vi "Servo_serial_mac_readwrite.vi"() -> ()   [LabVIEW 2017]
uses:
  <vilib>/Instr/_visa.llb/VISA Configure Serial Port (Instr).vi
panel:
  out "Servo 5 Position":cluster{i32, dbl, dbl[][]}(graph)
  out "Servo 4 Position":cluster{i32, dbl, dbl[][]}(graph)
  out "Servo 3 Position":cluster{i32, dbl, dbl[][]}(graph)
  out "Servo 2 Position":cluster{i32, dbl, dbl[][]}(graph)
  out "Servo 1 Position":cluster{i32, dbl, dbl[][]}(graph)
  out "Pos1 number":dbl
  out "Pos2 number":dbl
  out "Pos3 number":dbl
  out "Pos4 number":dbl
  out "Pos5 number":dbl
  in  "Delay":dbl
  in  "Buad Rate":i32(ring) items=["2400"=2400, "4800"=4800, "9600"=9600, "14400"=14400, "19200"=19200, "28800"=28800, "38400"=38400, "57600"=57600, "115200"=115200]
  out "Bytes at port":cluster{i32, dbl, dbl[]}(graph)
  out "Read from Arduino":string
  in  "Servo 5":dbl(knob) scale=0.0..180.0
  in  "Servo 4":dbl(knob) scale=0.0..180.0
  in  "Servo 3":dbl(knob) scale=0.0..180.0
  in  "Servo 2":dbl(knob) scale=0.0..180.0
  in  "Servo 1":dbl(knob) scale=0.0..180.0
  in  "stop":bool
  out "Sent to Arduino":string
  in  "COM Port":refnum<visa-resource-name>
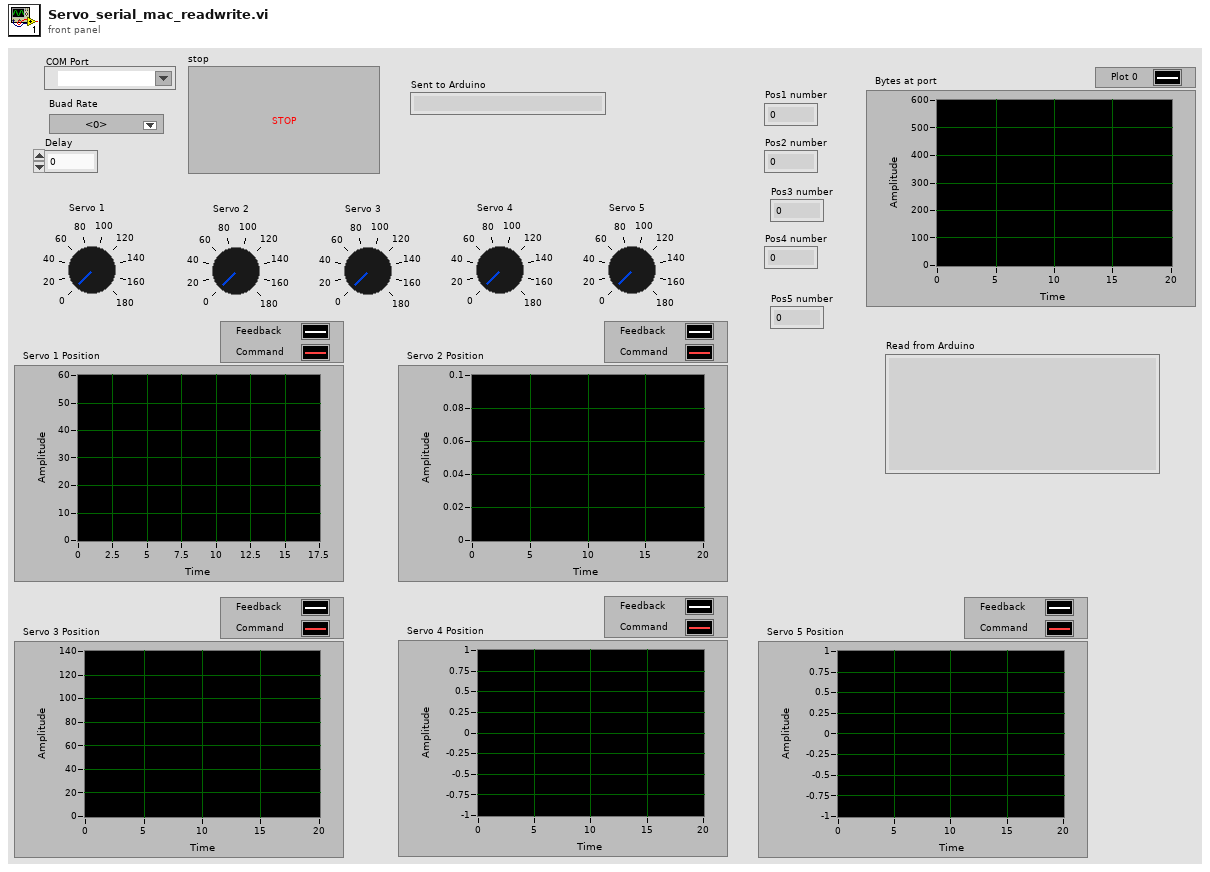
[diagram p1: front panel]
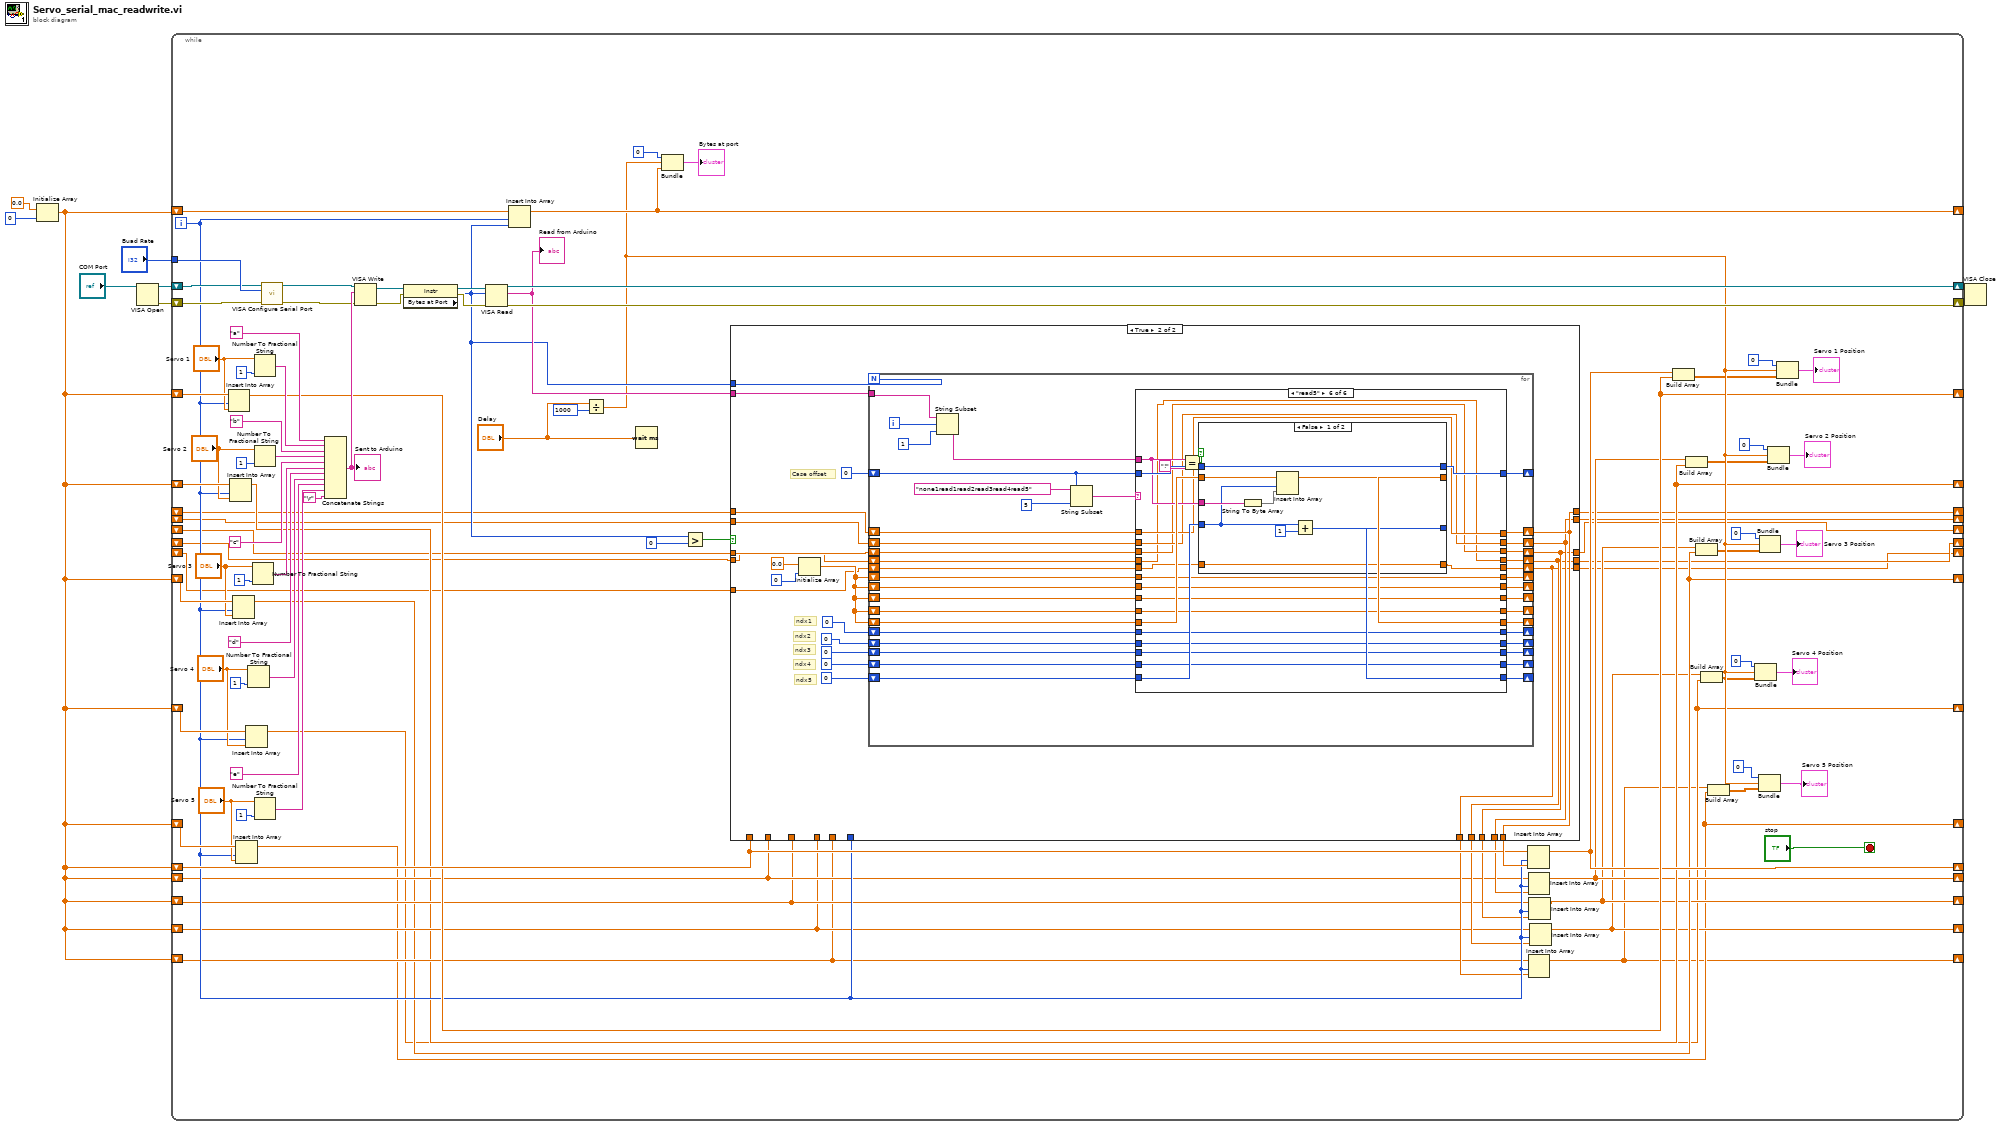
[diagram p0: block diagram]
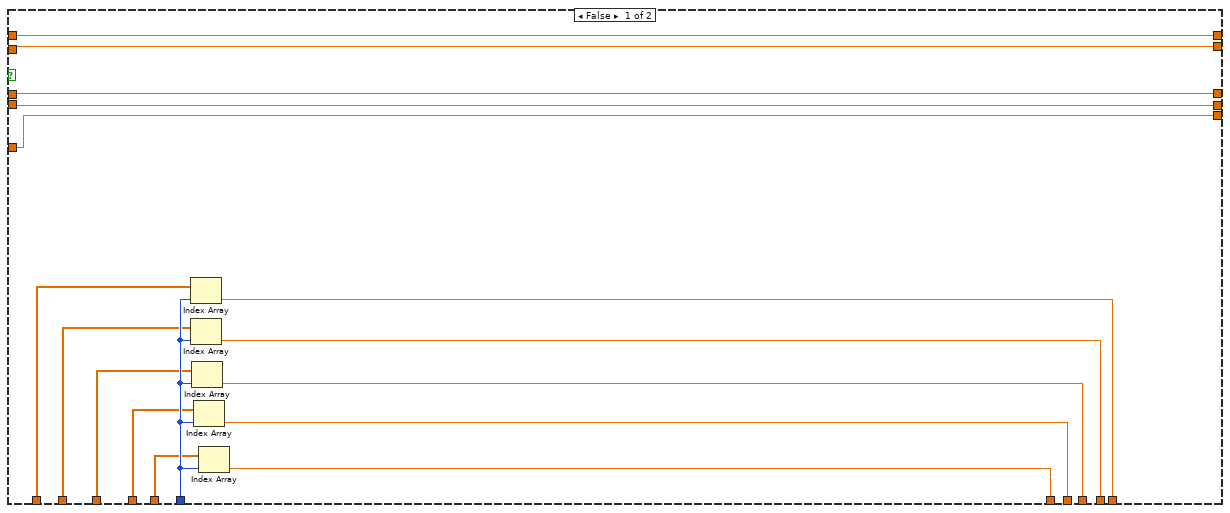
[diagram p2: hidden frame]
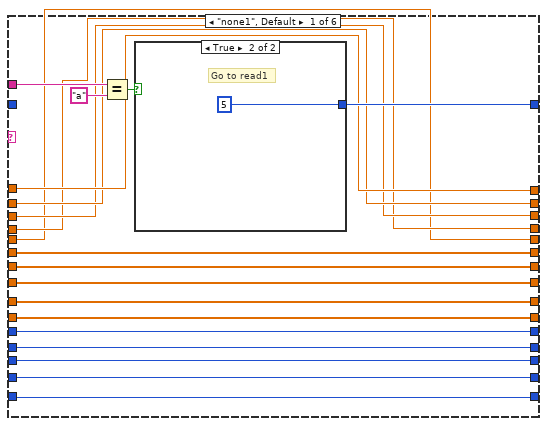
[diagram p3: hidden frame]
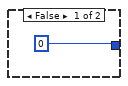
[diagram p4: hidden frame]
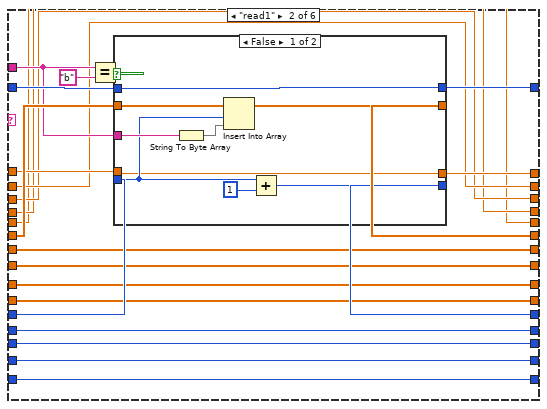
[diagram p5: hidden frame]
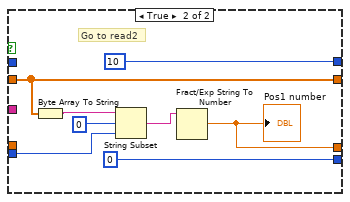
[diagram p6: hidden frame]
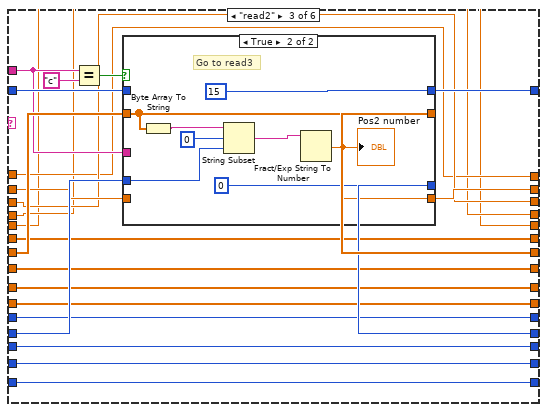
[diagram p7: hidden frame]
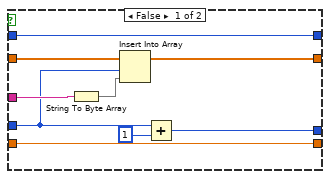
[diagram p8: hidden frame]
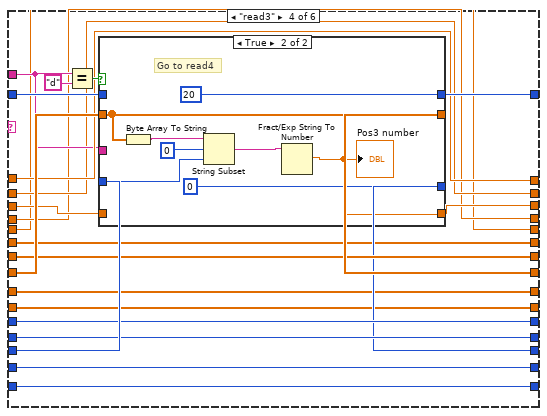
[diagram p9: hidden frame]
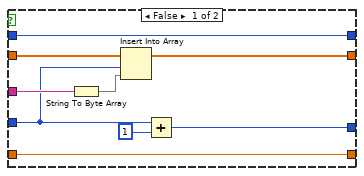
[diagram p10: hidden frame]
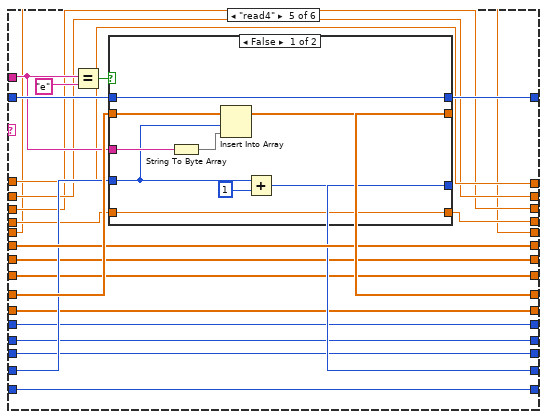
[diagram p11: hidden frame]
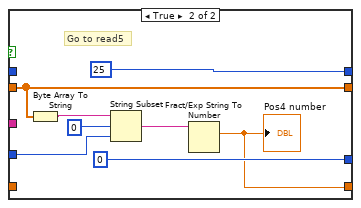
[diagram p12: hidden frame]
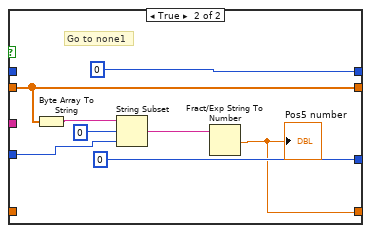
[diagram p13: hidden frame]
diagram:
  n1 = Initialize Array(0.0 ("element"), 0 ("dimension size")) -> (w1:dbl[])
  n2 = VISA Open(VISA resource name="COM Port") -> (VISA resource name=w8:refnum<visa-resource-name>, error out=w7:errorcluster)  [unwired: 4 in]
  n3 = while {
    tunnel: "Buad Rate" -> [w105]
    shift-right: [w101] -> w6
    shift-left: w8 -> [w104]
    shift-right: [w102] -> w5
    shift-left: w7 -> [w103]
    shift-right: [w99] -> _
    shift-left: w1 -> [w100]
    shift-right: [w43] -> _
    shift-left: w1 -> [w66]
    shift-right: [w30] -> _
    shift-left: w1 -> [w65]
    shift-right: [w27] -> _
    shift-left: w1 -> [w64]
    shift-right: [w24] -> _
    shift-left: w1 -> [w63]
    shift-right: [w21] -> _
    shift-left: w1 -> [w62]
    shift-right: [w41] -> _
    shift-left: w1 -> [w45]
    shift-right: [w29] -> _
    shift-left: w1 -> [w35]
    shift-right: [w26] -> _
    shift-left: w1 -> [w34]
    shift-right: [w23] -> _
    shift-left: w1 -> [w33]
    shift-right: [w20] -> _
    shift-left: w1 -> [w32]
    shift-right: [w18] -> _
    shift-left: _ -> [w19]
    shift-right: [w13] -> _
    shift-left: _ -> [w17]
    shift-right: [w12] -> _
    shift-left: _ -> [w16]
    shift-right: [w11] -> _
    shift-left: _ -> [w15]
    shift-right: [w10] -> _
    shift-left: _ -> [w14]
    i -> [w40]
    stop <- "stop" stop-if-true
    n4 = Insert Into Array(array=w66, index=w40, new element="Servo 1") -> (w43:dbl[])
    n5 = Insert Into Array(array=w65, index=w40, new element="Servo 2") -> (w30:dbl[])
    n6 = Insert Into Array(array=w64, index=w40, new element="Servo 3") -> (w27:dbl[])
    n7 = Insert Into Array(array=w62, index=w40, new element="Servo 5") -> (w21:dbl[])
    n8 = Insert Into Array(array=w63, index=w40, new element="Servo 4") -> (w24:dbl[])
    n9 = Number To Fractional String(number="Servo 4", precision (6)=1) -> (F-format string=w86:string)  [unwired: 2 in]
    n10 = Number To Fractional String(number="Servo 3", precision (6)=1) -> (F-format string=w93:string)  [unwired: 2 in]
    n11 = Number To Fractional String(number="Servo 1", precision (6)=1) -> (F-format string=w95:string)  [unwired: 2 in]
    n12 = Number To Fractional String(number="Servo 2", precision (6)=1) -> (F-format string=w94:string)  [unwired: 2 in]
    n13 = Number To Fractional String(number="Servo 5", precision (6)=1) -> (F-format string=w85:string)  [unwired: 2 in]
    n14 = call-poly "VISA Configure Serial Port"("VISA resource name"=w104, "baud rate (9600)"=w105, "error in (no error)"=w103) -> ("VISA resource name out"=w84:refnum<visa-resource-name>, "error out"=w96:errorcluster)  [unwired: 11 in]
    n15 = Concatenate Strings("a", w95, "b", w94, "c", w93, "d", w86, "e", w85, "\r") -> (w97:string)
    "Sent to Arduino" <- w97
    n16 = VISA Write(VISA resource name=w84, write buffer=w97, error in (no error)=w96) -> (VISA resource name out=w80:refnum<visa-resource-name>, error out=w83:errorcluster)  [unwired: 1 out]
    n17 = property class="Instr"(reference=w80, error in=w83) -> (reference out=w81:refnum<visa-resource-name>, error out=w82:errorcluster, "Bytes at Port"=w74:u32)
    n18 = VISA Read(VISA resource name=w81, byte count=w74, error in (no error)=w82) -> (VISA resource name out=w101:refnum<visa-resource-name>, read buffer=w76:string, error out=w102:errorcluster)  [unwired: 1 out]
    "Read from Arduino" <- w76
    n19 = Insert Into Array(array=w100, index=w40, new element=w74) -> (w99:dbl[])
    n20 = Divide(x="Delay", y=1000) -> (x/y=w44:dbl)
    n21 = Wait (ms)(milliseconds to wait="Delay") -> ()  [unwired: 1 out]
    n22 = Bundle(0, w44, w99) -> (→"Bytes at port":cluster{i32, dbl, dbl[]})  [unwired: 1 in]
    n23 = Greater?(x=w74, y=0) -> (0:w73:bool)
    n24 = case shown="True" w73 {
      tunnel: w74 -> [_ w132]
      tunnel: w76 -> [_ w142]
      tunnel: [w120 w130] -> w46
      tunnel: w40 -> [w119 _]
      tunnel: w45 -> [w121 _]
      tunnel: [w114 w125] -> w39
      tunnel: [w113 w124] -> w38
      tunnel: [w112 w123] -> w37
      tunnel: [w111 w122] -> w36
      tunnel: w35 -> [w118 _]
      tunnel: w34 -> [w117 _]
      tunnel: w33 -> [w116 _]
      tunnel: w32 -> [w115 _]
      tunnel: w19 -> [w110 w131]
      tunnel: [w110 w130] -> w18
      tunnel: w17 -> [w109 w129]
      tunnel: w16 -> [w108 w128]
      tunnel: w15 -> [w107 w127]
      tunnel: w14 -> [w106 w126]
      tunnel: [w109 w125] -> w13
      tunnel: [w108 w124] -> w12
      tunnel: [w107 w123] -> w11
      tunnel: [w106 w122] -> w10
      frame False {
        n25 = Index Array(array=w121, index=w119) -> (element=w120:dbl)
        n26 = Index Array(array=w118, index=w119) -> (element=w114:dbl)
        n27 = Index Array(array=w117, index=w119) -> (element=w113:dbl)
        n28 = Index Array(array=w116, index=w119) -> (element=w112:dbl)
        n29 = Index Array(array=w115, index=w119) -> (element=w111:dbl)
      }
      frame True {
        # "ndx5"
        # "ndx4"
        # "ndx3"
        # "ndx2"
        # "ndx1"
        # "Case offset"
        n30 = Initialize Array(0.0 ("element"), 0 ("dimension size")) -> (w135:dbl[])
        n31 = for {
          N: w132 -> [_]
          tunnel: w142 -> [w180]
          shift-right: [w176] -> _
          shift-left: 0 -> [w167]
          shift-right: [w175] -> _
          shift-left: 0 -> [w174]
          shift-right: [w172] -> _
          shift-left: w135 -> [w173]
          shift-right: [w170] -> _
          shift-left: w135 -> [w171]
          shift-right: [w163] -> _
          shift-left: 0 -> [w169]
          shift-right: [w164] -> _
          shift-left: 0 -> [w165]
          shift-right: [w161] -> _
          shift-left: w135 -> [w162]
          shift-right: [w153] -> _
          shift-left: w135 -> [w160]
          shift-right: [w154] -> _
          shift-left: w135 -> [w159]
          shift-right: [w157] -> _
          shift-left: 0 -> [w158]
          shift-right: [w155] -> _
          shift-left: 0 -> [w156]
          shift-right: [w152] -> w130
          shift-left: w131 -> [w151]
          shift-right: [w150] -> w125
          shift-left: w129 -> [w149]
          shift-right: [w148] -> w124
          shift-left: w128 -> [w147]
          shift-right: [w146] -> w123
          shift-left: w127 -> [w145]
          shift-right: [w144] -> w122
          shift-left: w126 -> [w143]
          i -> [w166]
          n32 = String Subset(string=w180, offset (0)=w166, length (rest)=1 ("length (rest)")) -> (substring=w177:string)
          n33 = String Subset(string="none1read1read2read3read4read5", offset (0)=w167, length (rest)=5 ("length (rest)")) -> (substring=w168:string)
          n34 = case shown="\"read5\"" w168 {
            tunnel: w177 -> [w200 w219 w255 w289 w338 w379]
            tunnel: [w197 w222 w257 w297 w345 w382] -> w176
            tunnel: [w196 w217 w259 w302 w335 w372] -> w175
            tunnel: w174 -> [w196 w218 w259 w302 w335 w372]
            tunnel: w173 -> [w193 w220 w254 w283 w342 w376]
            tunnel: [w193 w223 w254 w283 w342 w376] -> w172
            tunnel: w171 -> [w194 w216 w265 w298 w333 w375]
            tunnel: [w194 w216 w264 w298 w333 w375] -> w170
            tunnel: w169 -> [w195 w212 w263 w301 w334 w371]
            tunnel: [w195 w212 w262 w301 w334 w371] -> w163
            tunnel: w167 -> [_ w221 w258 w304 w339 w381]
            tunnel: w165 -> [w190 w211 w256 w303 w330 w370]
            tunnel: [w190 w211 w256 w294 w330 w370] -> w164
            tunnel: w162 -> [w187 w215 w253 w300 w332 w374]
            tunnel: [w187 w215 w253 w299 w332 w374] -> w161
            tunnel: w160 -> [w188 w214 w252 w293 w344 w373]
            tunnel: w159 -> [w189 w213 w251 w292 w331 w384]
            tunnel: w158 -> [w192 w210 w250 w296 w337 w369]
            tunnel: [w192 w210 w250 w296 w336 w369] -> w157
            tunnel: w156 -> [w191 w209 w249 w295 w329 w378]
            tunnel: [w191 w209 w249 w295 w329 w377] -> w155
            tunnel: [w189 w213 w251 w292 w331 w383] -> w154
            tunnel: [w188 w214 w252 w293 w343 w373] -> w153
            tunnel: [w186 w208 w245 w291 w328 w368] -> w152
            tunnel: w151 -> [w186 w207 w245 w291 w328 w368]
            tunnel: [w185 w206 w248 w288 w327 w367] -> w150
            tunnel: w149 -> [w185 w206 w247 w288 w327 w367]
            tunnel: [w184 w205 w246 w287 w324 w365] -> w148
            tunnel: w147 -> [w184 w205 w246 w286 w324 w365]
            tunnel: [w183 w204 w244 w285 w326 w363] -> w146
            tunnel: w145 -> [w183 w204 w244 w285 w325 w363]
            tunnel: [w182 w203 w243 w284 w323 w366] -> w144
            tunnel: w143 -> [w182 w203 w243 w284 w323 w364]
            frame "none1", Default {
              n35 = Equal?(x=w200, y="a") -> (x = y?=w198:bool)
              n36 = case shown="True" w198 {
                tunnel: [0 5] -> w197
                frame False {
                }
                frame True {
                  # "Go to read1"
                }
              }
            }
            frame "read1" {
              n37 = Equal?(x=w219, y="b") -> (x = y?=w224:bool)
              n38 = case shown="False" w224 {
                tunnel: [w234 0] -> w217
                tunnel: w220 -> [w228 w238]
                tunnel: [w232 w238] -> w223
                tunnel: w219 -> [w231 _]
                tunnel: [w229 10] -> w222
                tunnel: w221 -> [w229 _]
                tunnel: w218 -> [w227 w237]
                tunnel: [w226 w235] -> w208
                tunnel: w207 -> [w226 _]
                frame False {
                  n39 = String To Byte Array(string=w231) -> (unsigned byte array=w230:u8[])
                  n40 = Insert Into Array(array=w228, index=w227, new element=w230) -> (w232:dbl[])
                  n41 = Add(x=w227, y=1) -> (x+y=w234:i32)
                }
                frame True {
                  # "Go to read2"
                  n42 = Byte Array To String(unsigned byte array=w238) -> (string=w239:string)
                  n43 = String Subset(string=w239, offset (0)=0, length (rest)=w237) -> (substring=w236:string)
                  n44 = Fract/Exp String To Number(string=w236) -> (number=w235:dbl)  [unwired: 3 in, 1 out]
                  "Pos1 number" <- w235
                }
              }
            }
            frame "read2" {
              n45 = Equal?(x=w255, y="c") -> (x = y?=w260:bool)
              n46 = case shown="True" w260 {
                tunnel: [w274 0] -> w262
                tunnel: w263 -> [w268 w279]
                tunnel: w265 -> [w272 w278]
                tunnel: [w271 w278] -> w264
                tunnel: w255 -> [w270 _]
                tunnel: [w267 15] -> w257
                tunnel: w258 -> [w267 _]
                tunnel: [w266 w275] -> w248
                tunnel: w247 -> [w266 _]
                frame False {
                  n47 = String To Byte Array(string=w270) -> (unsigned byte array=w269:u8[])
                  n48 = Insert Into Array(array=w272, index=w268, new element=w269) -> (w271:dbl[])
                  n49 = Add(x=w268, y=1) -> (x+y=w274:i32)
                }
                frame True {
                  # "Go to read3"
                  n50 = Byte Array To String(unsigned byte array=w278) -> (string=w277:string)
                  n51 = String Subset(string=w277, offset (0)=0, length (rest)=w279) -> (substring=w276:string)
                  n52 = Fract/Exp String To Number(string=w276) -> (number=w275:dbl)  [unwired: 3 in, 1 out]
                  "Pos2 number" <- w275
                }
              }
            }
            frame "read3" {
              n53 = Equal?(x=w289, y="d") -> (x = y?=w305:bool)
              n54 = case shown="True" w305 {
                tunnel: [w314 0] -> w294
                tunnel: w303 -> [w308 w317]
                tunnel: w300 -> [w312 w318]
                tunnel: [w311 w318] -> w299
                tunnel: w289 -> [w310 _]
                tunnel: [w307 20] -> w297
                tunnel: w304 -> [w307 _]
                tunnel: [w306 w315] -> w287
                tunnel: w286 -> [w306 _]
                frame False {
                  n55 = String To Byte Array(string=w310) -> (unsigned byte array=w309:u8[])
                  n56 = Insert Into Array(array=w312, index=w308, new element=w309) -> (w311:dbl[])
                  n57 = Add(x=w308, y=1) -> (x+y=w314:i32)
                }
                frame True {
                  # "Go to read4"
                  n58 = Byte Array To String(unsigned byte array=w318) -> (string=w319:string)
                  n59 = String Subset(string=w319, offset (0)=0, length (rest)=w317) -> (substring=w316:string)
                  n60 = Fract/Exp String To Number(string=w316) -> (number=w315:dbl)  [unwired: 3 in, 1 out]
                  "Pos3 number" <- w315
                }
              }
            }
            frame "read4" {
              n61 = Equal?(x=w338, y="e") -> (x = y?=w340:bool)
              n62 = case shown="False" w340 {
                tunnel: [w354 0] -> w336
                tunnel: w337 -> [w348 w357]
                tunnel: w344 -> [w352 w358]
                tunnel: [w351 w358] -> w343
                tunnel: w338 -> [w350 _]
                tunnel: [w347 25] -> w345
                tunnel: w339 -> [w347 _]
                tunnel: [w346 w355] -> w326
                tunnel: w325 -> [w346 _]
                frame False {
                  n63 = String To Byte Array(string=w350) -> (unsigned byte array=w349:u8[])
                  n64 = Insert Into Array(array=w352, index=w348, new element=w349) -> (w351:dbl[])
                  n65 = Add(x=w348, y=1) -> (x+y=w354:i32)
                }
                frame True {
                  # "Go to read5"
                  n66 = Byte Array To String(unsigned byte array=w358) -> (string=w359:string)
                  n67 = String Subset(string=w359, offset (0)=0, length (rest)=w357) -> (substring=w356:string)
                  n68 = Fract/Exp String To Number(string=w356) -> (number=w355:dbl)  [unwired: 3 in, 1 out]
                  "Pos4 number" <- w355
                }
              }
            }
            frame "read5" {
              n69 = Equal?(x=w379, y="!") -> (x = y?=w380:bool)
              n70 = case shown="False" w380 {
                tunnel: [w394 0] -> w377
                tunnel: w378 -> [w388 w397]
                tunnel: w384 -> [w392 w398]
                tunnel: [w391 w398] -> w383
                tunnel: w379 -> [w390 _]
                tunnel: [w387 0] -> w382
                tunnel: w381 -> [w387 _]
                tunnel: [w386 w395] -> w366
                tunnel: w364 -> [w386 _]
                frame False {
                  n71 = String To Byte Array(string=w390) -> (unsigned byte array=w389:u8[])
                  n72 = Insert Into Array(array=w392, index=w388, new element=w389) -> (w391:dbl[])
                  n73 = Add(x=w388, y=1) -> (x+y=w394:i32)
                }
                frame True {
                  # "Go to none1"
                  n74 = Byte Array To String(unsigned byte array=w398) -> (string=w399:string)
                  n75 = String Subset(string=w399, offset (0)=0, length (rest)=w397) -> (substring=w396:string)
                  n76 = Fract/Exp String To Number(string=w396) -> (number=w395:dbl)  [unwired: 3 in, 1 out]
                  "Pos5 number" <- w395
                }
              }
            }
          }
        }
      }
    }
    n77 = Insert Into Array(array=w45, index=w40, new element=w46) -> (w41:dbl[])
    n78 = Insert Into Array(array=w35, index=w40, new element=w39) -> (w29:dbl[])
    n79 = Insert Into Array(array=w32, index=w40, new element=w36) -> (w20:dbl[])
    n80 = Insert Into Array(array=w34, index=w40, new element=w38) -> (w26:dbl[])
    n81 = Insert Into Array(array=w33, index=w40, new element=w37) -> (w23:dbl[])
    n82 = Build Array(w41, w43) -> (w42:dbl[][])
    n83 = Build Array(w29, w30) -> (w31:dbl[][])
    n84 = Build Array(w26, w27) -> (w28:dbl[][])
    n85 = Build Array(w23, w24) -> (w25:dbl[][])
    n86 = Build Array(w20, w21) -> (w22:dbl[][])
    n87 = Bundle(0, w44, w25) -> (→"Servo 4 Position":cluster{i32, dbl, dbl[][]})  [unwired: 1 in]
    n88 = Bundle(0, w44, w22) -> (→"Servo 5 Position":cluster{i32, dbl, dbl[][]})  [unwired: 1 in]
    n89 = Bundle(0, w44, w28) -> (→"Servo 3 Position":cluster{i32, dbl, dbl[][]})  [unwired: 1 in]
    n90 = Bundle(0, w44, w31) -> (→"Servo 2 Position":cluster{i32, dbl, dbl[][]})  [unwired: 1 in]
    n91 = Bundle(0, w44, w42) -> (→"Servo 1 Position":cluster{i32, dbl, dbl[][]})  [unwired: 1 in]
  }
  n92 = VISA Close(VISA resource name=w6, error in (no error)=w5) -> ()  [unwired: 1 out]
